vi "action.vi"(0 "MoAgSy_Engine":refnum<class "MoAgSy_Engine.lvclass">, 5 "error in":errorcluster, 8 "HGF_ThreadWorker":refnum<class "HGF_ThreadWorker.lvclass">) -> (10 "dup HGF_ThreadWorker":refnum<class "HGF_ThreadWorker.lvclass">, 14 "dup MoAgSy_Engine":refnum<class "MoAgSy_Engine.lvclass">, 19 "error out":errorcluster)   [LabVIEW 2009, in "MoAgSy.lvlib" / "MoAgSy_Engine.lvclass"]
uses:
  MoAgSy_Engine.lvclass
  HGF_BaseClasses/HGF_ThreadWorker/HGF_ThreadWorker.lvclass
  MoAgSy_StateMachine/MoAgSy_StateMachine.lvsc/StatechartState.ctl
  MoAgSy_StateMachine/MoAgSy_StateMachine.lvsc/State.ctl
  MoAgSy_StateMachine/MoAgSy_StateMachine.lvsc/Inputs.ctl
  MoAgSy_AgentBase/MoAgSy_AgentBase.lvclass
  HGF_BaseClasses/HGF_Event/HGF_Event.lvclass
  MoAgSy_StateMachine/MoAgSy_StateMachine.lvsc/Trigger.ctl
  MoAgSy_Engine.lvclass/MoAgSy_Engine.ctl
  <vilib>/Statechart/Infrastructure/RTStatechart/RunTime SCN.xnode
  MoAgSy_StateMachine/MoAgSy_StateMachine.lvsc/CompanionDiagram.vi/66/SC Main.vi
  <vilib>/Statechart/Common/IntGuid.ctl
  <vilib>/Statechart/Common/DbgID.ctl
  MoAgSy_StateMachine/MoAgSy_StateMachine.lvsc
  MoAgSy_StateMachine/MoAgSy_StateMachine.lvsc/Outputs.ctl
  Visitors/MoAgSy_Visitor/MoAgSy_Visitor.lvclass
  <vilib>/Statechart/Common/NI_SC_LVSCCommonFiles.lvlib
panel:
  out "Worker Stop Error":bool
  out "Active States":T1
  out "Agent ID":string
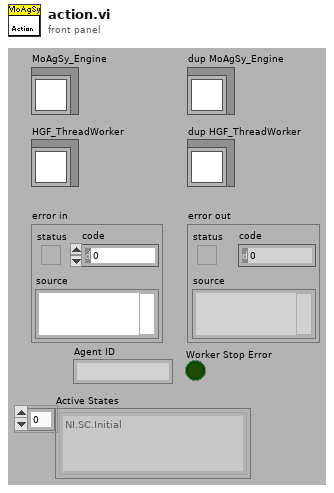
[diagram p1: front panel]
types:
  T1 = typedef "MoAgSy.lvlib/MoAgSy_StateMachine.lvsc/StatechartState.ctl" = T2[]
  T2 = typedef "MoAgSy.lvlib/MoAgSy_StateMachine.lvsc/State.ctl" = enum16{"NI.SC.Initial", "NI.SC.History", "NI.SC.ShallowHistory", "NI.SC.Terminal", "shutdown", "travel", "init", "Running", "Running\\Running states\\handle Event", "Running\\Running states\\waiting", "Running\\Running states\\handle Event\\EventHandling\\mobile Agent", "Running\\Running states\\handle Event\\EventHandling\\msg handler", "Running\\Running states\\handle Event\\EventHandling\\visitor", "Running\\Running states\\handle Event\\EventHandling\\send msg", "Running\\Running states\\handle Event\\EventHandling\\get\nReceiver\n&\nType"}
  T3 = typedef "MoAgSy.lvlib/MoAgSy_StateMachine.lvsc/Trigger.ctl" = enum16{"NULL", "initialized", "Error", "Shutdown", "Event", "Reset", "Ready", "reply", "visitor", "msg", "MoAg", "travel"}
  T4 = typedef "MoAgSy.lvlib/MoAgSy_StateMachine.lvsc/Inputs.ctl" = cluster{"HGF_Agent":refnum<class "MoAgSy_AgentBase.lvclass">, "HGF_Event (Monitor Event)":refnum<class "HGF_Event.lvclass">, "Incoming":refnum<class>, "VarManagerEvent":refnum<class "HGF_Event.lvclass">}
  T5 = typedef "NI_SC_LVSCCommonFiles.lvlib/IntGuid.ctl" = cluster{"Data1":u32, "Data2":u16, "Data3":u16, "Data4":u8, "Data5":u8, "Data6":u8, "Data11":u8, "Data9":u8, "Data10":u8, "Data8":u8, "Data7":u8}
  T6 = typedef "NI_SC_LVSCCommonFiles.lvlib/DbgID.ctl" = cluster{"VIRef":u32, "IntGUID":T5}
  T7 = typedef "MoAgSy.lvlib/MoAgSy_StateMachine.lvsc/Outputs.ctl" = cluster{"Numeric":i8, "Agent ID":string, "Trigger":T3, "int Trigger?":bool, "error out":errorcluster, "Destination":string, "Event Array":refnum<class "HGF_Event.lvclass">[], "standard Visitor":cluster{"Standard Visitor":refnum<class "MoAgSy_Visitor.lvclass">, "timeout":dbl}}
  T8 = cluster{"Standard Visitor":refnum<class "MoAgSy_Visitor.lvclass">, "timeout":dbl}
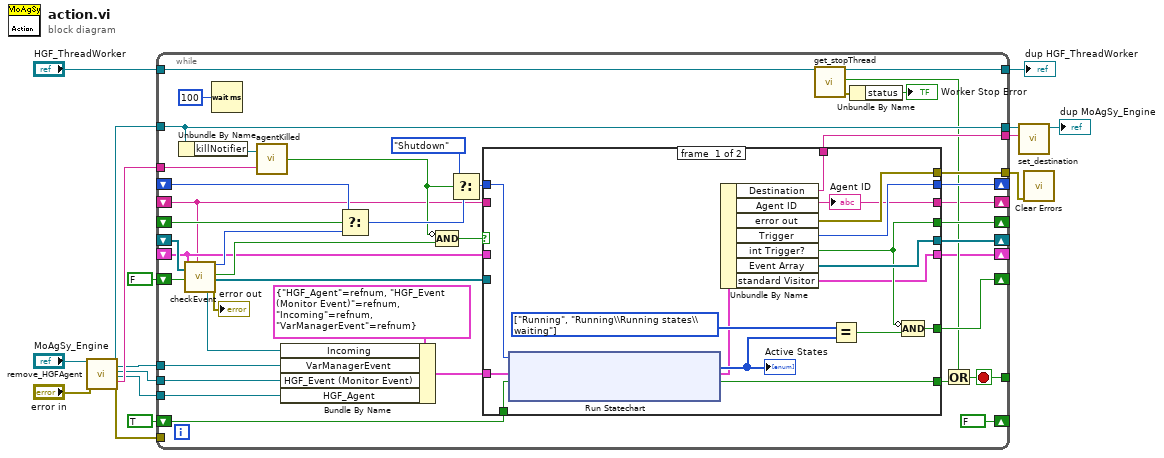
[diagram p0: block diagram]
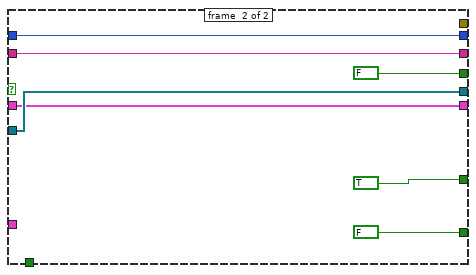
[diagram p2: hidden frame]
diagram:
  n1 = call "remove_HGFAgent.vi"("MoAgSy_Engine.lvclass in"="MoAgSy_Engine", "error in (no error)"="error in") -> ("MoAgSy_Engine.lvclass out"=w14:refnum<class "MoAgSy_Engine.lvclass">, "VarManagerEvent"=w4:refnum<class "HGF_Event.lvclass">, "HGF_Event (Monitor Event)"=w5:refnum<class "HGF_Event.lvclass">, "HGF_Agent"=w6:refnum<class "MoAgSy_AgentBase.lvclass">, "Agent ID"=w7:string, "error out"=w12:errorcluster)  [unwired: 12 out]
  n2 = while {
    tunnel: "HGF_ThreadWorker" -> [w28]
    tunnel: [w27] -> w15
    tunnel: w14 -> [w57]
    tunnel: [w57] -> w11
    tunnel: w12 -> [_]
    tunnel: w6 -> [w53]
    tunnel: [w26] -> _
    tunnel: w7 -> [w58]
    shift-right: [w35] -> _
    shift-left: _ -> [w48]
    shift-right: [w36] -> _
    shift-left: _ -> [w47]
    shift-right: [FALSE] -> _
    shift-left: TRUE -> [w45]
    tunnel: w5 -> [w44]
    tunnel: w4 -> [w43]
    tunnel: [w34] -> w1
    tunnel: [w33] -> w3
    shift-right: [w42] -> _
    shift-left: FALSE -> [w40]
    shift-right: [w37] -> _
    shift-left: _ -> [w41]
    shift-right: [w23] -> _
    shift-left: _ -> [w22]
    shift-right: [w21] -> _
    shift-left: _ -> [w20]
    stop <- w26 stop-if-true
    n3 = Unbundle By Name(w57) -> ("killNotifier"=w55:refnum<notifier>)
    n4 = call "checkEvent.vi"("standard Visitor"=w22, "Event Array"=w41, "Status on event?"=w40, "Agent ID"=w20) -> ("Object"=w39:refnum<class>, "Event/Null"=w38:T3, "timed out"=w32:bool, "dup Event Array"=w31:refnum<class "HGF_Event.lvclass">[], "error out"=→"error out":errorcluster)  [unwired: 11 out]
    n5 = Wait (ms)(milliseconds to wait=u32 100) -> ()  [unwired: 1 out]
    n6 = call "agentKilled.vi"("Agent ID"=w58, "killNotifier"=w55) -> ("Stop"=w30:bool)
    n7 = Bundle By Name(cluster=T4 {"HGF_Agent"=refnum, "HGF_Event (Monitor Event)"=refnum, "Incoming"=refnum, "VarManagerEvent"=refnum} ("Inputs"), "Incoming"=w39, "VarManagerEvent"=w43, "HGF_Event (Monitor Event)"=w44, "HGF_Agent"=w53) -> (w52:T4)
    n8 = Select(t=w48, s=w47, f=w38) -> (s? t:f=w49:T3)
    n9 = Compound Arithmetic op=AND(invert w30, w32) -> (w29:bool)
    n10 = Select(t=Trigger."Shutdown" ("Trigger"), s=w30, f=w49) -> (s? t:f=w50:T3)
    n11 = case shown="False" w29 {
      tunnel: w52 -> [w74 _]
      tunnel: w50 -> [w64 w178]
      tunnel: [w73 FALSE ("Terminated?")] -> w25
      tunnel: w45 -> [w72 _]
      tunnel: [w63 TRUE] -> w42
      tunnel: w31 -> [_ w177]
      tunnel: [w68 w177] -> w37
      tunnel: [w62 FALSE ("int Trigger?")] -> w36
      tunnel: [w67 w178] -> w35
      tunnel: [w65 _] -> w34
      tunnel: [w66 _] -> w33
      tunnel: [w61 w173] -> w23
      tunnel: w22 -> [_ w173]
      tunnel: [w60 w172] -> w21
      tunnel: w20 -> [_ w172]
      frame #0 {
        n12 = xnode "Run Statechart"("Init?"=w72, "Inputs"=w74, "Trigger"=w64) -> ("Terminated?"=w73:bool, "Outputs"=w59:T7, "Active States"=w71:T1)
        "Active States" <- w71
        n13 = Unbundle By Name(w59) -> ("Destination"=w66:string, "Agent ID"=w60:string, "error out"=w65:errorcluster, "Trigger"=w67:T3, "int Trigger?"=w62:bool, "Event Array"=w68:refnum<class "HGF_Event.lvclass">[], "standard Visitor"=w61:T8)
        "Agent ID" <- w60
        n14 = Equal?(x=T1 [enum."Running", enum."Running\\Running states\\waiting"] ("Active States"), y=w71) -> (x = y?=w69:bool)
        n15 = Compound Arithmetic op=AND(invert w62, w69) -> (w63:bool)
      }
      frame #1 {
      }
    }
    n16 = call "get_stopThread.vi"("HGF_ThreadWorker"=w28) -> ("dup HGF_ThreadWorker"=w27:refnum<class "HGF_ThreadWorker.lvclass">, "stopThread"=w24:bool, "error out"=w19:errorcluster)  [unwired: 16 in]
    n17 = Unbundle By Name(w19) -> ("status"=→"Worker Stop Error":bool)
    n18 = Or(x=w24, y=w25) -> (x .or. y?=w26:bool)
  }
  "dup HGF_ThreadWorker" <- w15
  n19 = call "set_destination.vi"("destination"=w3, "MoAgSy_Engine.lvclass in"=w11) -> ("MoAgSy_Engine.lvclass out"=→"dup MoAgSy_Engine":refnum<class "MoAgSy_Engine.lvclass">)  [unwired: 1 in, 8 out]
  n20 = call <vilib>:"Clear Errors.vi"("error in (no error)"=w1) -> ()  [unwired: 6 in, 1 out]
